vi "Feedback node testing.vi"() -> ()   [LabVIEW 2018]
panel:
  in  "停止":bool
  out "x-y":dbl
  out "数值 2":dbl
  out "数值":i32
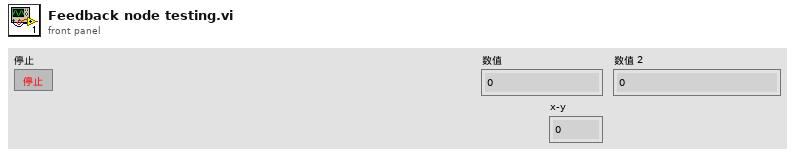
[diagram p1: front panel]
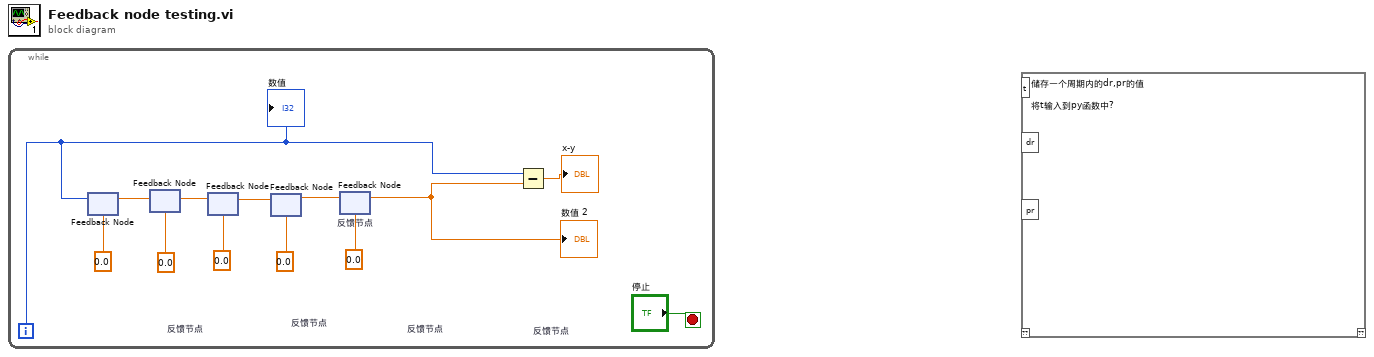
[diagram p0: block diagram]
diagram:
  n1 = while {
    i -> [w12]
    stop <- "停止" stop-if-true
    n2 = feedback #1 "反馈节点"(0.0) -> (w9:dbl)
    n3 = feedback-in #1(w12) -> ()
    n4 = feedback #2 "反馈节点"(0.0) -> (w7:dbl)
    n5 = feedback-in #2(w9) -> ()
    n6 = feedback #3 "反馈节点"(0.0) -> (w4:dbl)
    n7 = feedback-in #3(w7) -> ()
    n8 = feedback #4 "反馈节点"(0.0) -> (w2:dbl)
    n9 = feedback-in #4(w4) -> ()
    n10 = feedback #5 "反馈节点"(0.0) -> (w1:dbl)
    "数值 2" <- w1
    n11 = feedback-in #5(w2) -> ()
    n12 = Subtract(x=w12, y=w1) -> (x-y=→"x-y":dbl)
    "数值" <- w12
  }
  n13 = script code="储存一个周期内的dr,pr的值\n\n将t输入到py函数中?"() -> ()  [unwired: 4 in, 1 out]
